vi "Close.vi"(8 "error in (no error)":errorcluster, 11 "Log Sinks in":refnum<class "Log Sinks.lvclass">) -> (0 "error out":errorcluster, 3 "Log Sinks out":refnum<class "Log Sinks.lvclass">)   [LabVIEW 2019, in "TSC Event Logger.lvlib" / "Log Sinks.lvclass"]
uses:
  Log Sinks.lvclass
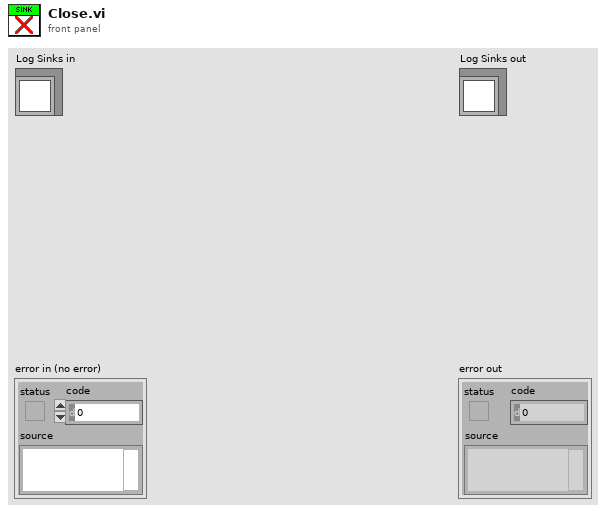
[diagram p1: front panel]
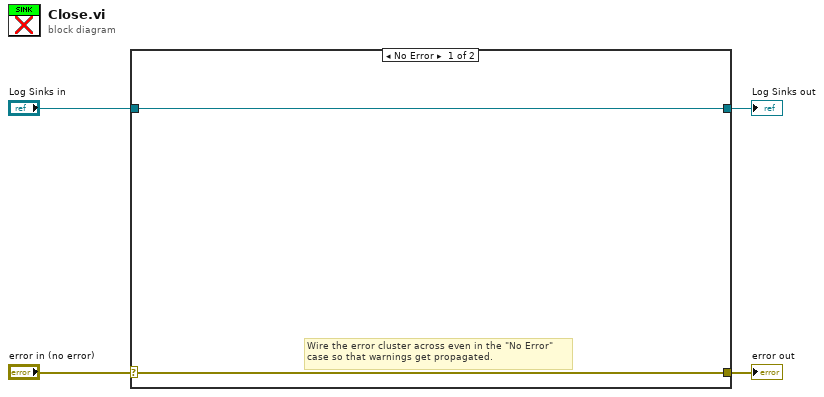
[diagram p0: block diagram]
diagram:
  n1 = case shown="No Error" "error in (no error)" {
    selector: "error in (no error)" -> [w5 w8]
    tunnel: [w5 w8] -> w3
    tunnel: [w6 w7] -> w1
    tunnel: "Log Sinks in" -> [w6 w7]
    frame No Error {
      # "Wire the error cluster across even in the \"No Error\"\ncase so that warnings get propagated."
    }
    frame Error {
    }
  }
  "error out" <- w3
  "Log Sinks out" <- w1
